vi "Wavelength Meter (No Objects).vi"(8 "error in (no error)":errorcluster, 11 "Cluster In":T3={"Exp Range Min"=0, "Exp Range Max"=0, "exposure mode"=enum."manual", "operation (meas. mode)"=enum."Measurement mode", "Exposure (ms)"=0, "Quiet Errors?"=FALSE, "Error Status"={"status"=FALSE, "code"=0, "source"=""}}) -> (0 "error out":errorcluster, 3 "Cluster Out":T3={"Exp Range Min"=0, "Exp Range Max"=0, "exposure mode"=enum."manual", "operation (meas. mode)"=enum."Measurement mode", "Exposure (ms)"=0, "Quiet Errors?"=FALSE, "Error Status"={"status"=FALSE, "code"=0, "source"=""}})   [LabVIEW 2009]
uses:
  HighFinesse WS5/Variable Typedefs.llb/Exposure Mode.ctl
  HighFinesse WS5/Control typedefs.llb/Measurement Mode.ctl
  <vilib>/Utility/error.llb/DialogType.ctl
  HighFinesse WS5/Variable Typedefs.llb/WLM control mode.ctl
  HighFinesse WS5/HighFinesse WS5.lvlib
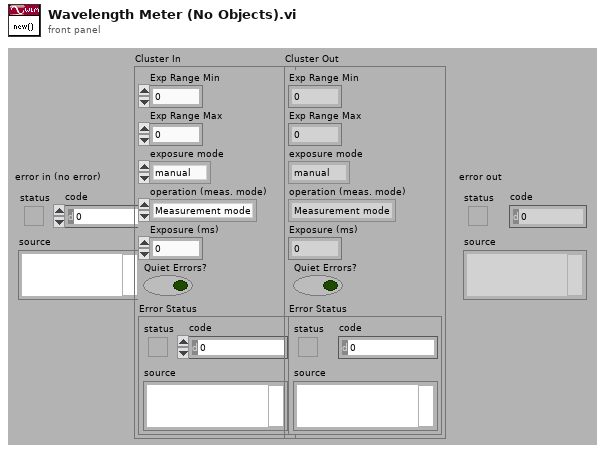
[diagram p1: front panel]
types:
  T1 = typedef "HighFinesse WS5.lvlib/Exposure Mode.ctl" = enum16{"manual", "automatic"}
  T2 = typedef "HighFinesse WS5.lvlib/Measurement Mode.ctl" = enum16{"Measurement off", "Adjustment mode", "Measurement mode"}
  T3 = cluster{"Exp Range Min":u32, "Exp Range Max":u32, "exposure mode":T1, "operation (meas. mode)":T2, "Exposure (ms)":u16, "Quiet Errors?":bool, "Error Status":errorcluster}
  T4 = typedef "DialogType.ctl" = u16
  T5 = typedef "HighFinesse WS5.lvlib/WLM control mode.ctl" = i16
  T6 = enum16{"Measurement off", "Adjustment mode", "Measurement mode"}
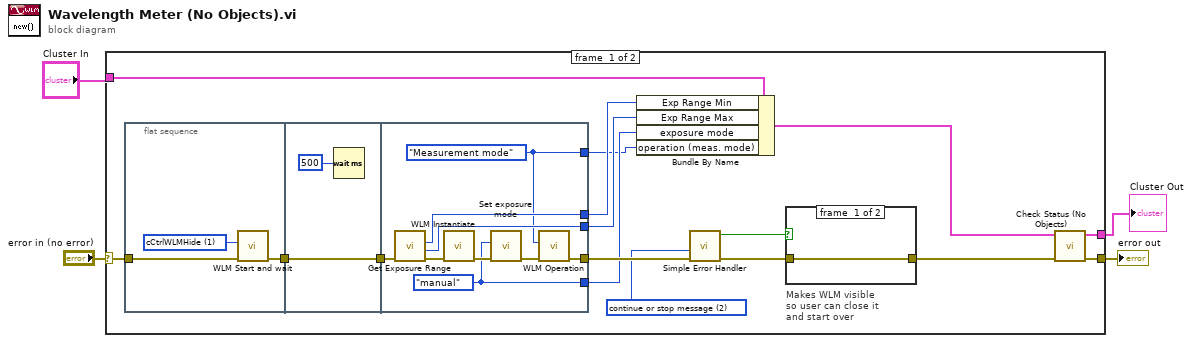
[diagram p0: block diagram]
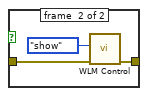
[diagram p2: hidden frame]
diagram:
  n1 = case shown="No Error" "error in (no error)" {
    selector: "error in (no error)" -> [w20 w40]
    tunnel: [w14 w40] -> w3
    tunnel: [w13 w39] -> w1
    tunnel: "Cluster In" -> [w17 w39]
    frame #0 {
      w11 = T4 2 items=["no dialog", "OK message", "continue or stop message", "OK message + warnings", "continue/stop + warnings"] ("type of dialog (OK msg:1)")
      n2 = flat-sequence {
        tunnel: w20 -> [w27]
        tunnel: [w26] -> w18
        tunnel: [w28] -> w19
        tunnel: w18 -> [w28]
        tunnel: [w36] -> w12
        tunnel: w19 -> [w35]
        tunnel: [w33] -> w16
        tunnel: [w32] -> w15
        tunnel: [w31] -> w10
        tunnel: [w30] -> w9
        frame #0 {
          w25 = T5 1 items=["cCtrlWLMShow", "cCtrlWLMHide", "cCtrlWLMExit"] ("WLM Control Mode Constants")
          n3 = call "WLM Start and wait.vi"("error in (no error)"=w27, "WLM Control Mode Constants"=w25) -> ("error out"=w26:errorcluster)  [unwired: 9 out]
        }
        frame #1 {
          n4 = Wait (ms)(milliseconds to wait=u32 500) -> ()  [unwired: 1 out]
        }
        frame #2 {
          w31 = Exposure_Mode."manual" ("exposure mode")
          w30 = T6."Measurement mode" ("operation (meas. mode)")
          n5 = call "Get Exposure Range.vi"("error in (no error)"=w35) -> ("error out"=w34:errorcluster, "Exp Range Max"=w32:u32, "Exp Range Min"=w33:u32)  [unwired: 8 in]
          n6 = call "WLM Instantiate.vi"("error in (no error)"=w34) -> ("error out"=w38:errorcluster)  [unwired: 9 in, 1 out]
          n7 = call "Set exposure mode.vi"("error in (no error)"=w38, "exposure mode"=w31) -> ("error out"=w37:errorcluster)  [unwired: 9 out]
          n8 = call "WLM Operation.vi"("error in (no error)"=w37, "operation (meas. mode)"=w30) -> ("error out"=w36:errorcluster)  [unwired: 9 out]
        }
      }
      n9 = Bundle By Name(cluster=w17, "Exp Range Min"=w16, "Exp Range Max"=w15, "exposure mode"=w10, "operation (meas. mode)"=w9) -> (w6:T3)
      n10 = call <vilib>:"Simple Error Handler.vi"("type of dialog (OK msg:1)"=w11, "error in (no error)"=w12) -> ("error?"=w8:bool, "error out"=w7:errorcluster)  [unwired: 3 in, 3 out]
      n11 = case "Makes WLM visible\nso user can close it\nand start over" shown="True" w8 {
        tunnel: w7 -> [w21 w23]
        tunnel: [w21 w22] -> w5
        frame #0 {
        }
        frame #1 {
          n12 = call "WLM Control.vi"("error in (no error)"=w23, "command"=enum16{"show", "hide", "exit"}."show") -> ("error out"=w22:errorcluster)  [unwired: 9 out]
        }
      }
      n13 = call "Check Status (No Objects).vi"("error in (no error)"=w5, "Cluster In"=w6) -> ("error out"=w14:errorcluster, "Cluster Out"=w13:T3)  [unwired: 6 in, 2 out]
    }
    frame #1 {
    }
  }
  "error out" <- w3
  "Cluster Out" <- w1
